vi "TDMS Advanced - Write Synchronously.vi"   [LabVIEW 2020]
panel:
  # "For instructions, select Help>>Show Context Help and move the cursor over the VI icon to display help for this VI."
types:
  T1 = enum16{"open", "open or create", "create or replace", "create", "open (read-only)"}
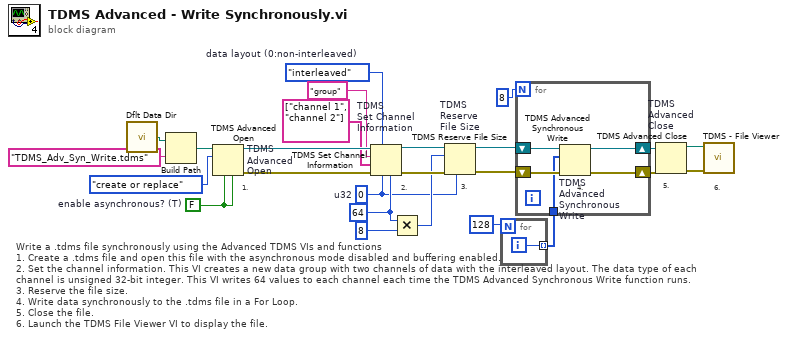
[diagram p0: block diagram]
diagram:
  w3 = FALSE  # enable asynchronous? (T)
  w7 = u32 64 ("samples per channel")
  w4 = u32 0  # u32
  w17 = enum16{"non-interleaved", "interleaved"}."interleaved"  # data layout (0:non-interleaved)
  # "Write a .tdms file synchronously using the Advanced TDMS VIs and functions\n1. Create a .tdms file and open this file with the asynchronous mode disabled and buffering enabled.\n2. Set the channel information. This VI creates a new data group with two channels of data with the interleaved layout. The data type of each channel is unsigned 32-bit integer. This VI writes 64 values to each channel each time the TDMS Advanced Synchronous Write function runs.\n3. Reserve the file size.\n4. Write data synchronously to the .tdms file in a For Loop.\n5. Close the file.\n6. Launch the TDMS File Viewer VI to display the file."
  # "6."
  # "1."
  # "5."
  # "3."
  # "2."
  n1 = call <vilib>:"Dflt Data Dir.vi"() -> ("App:Default Data Directory"=w20:path)
  n2 = Build Path(base path=w20, name or relative path="TDMS_Adv_Syn_Write.tdms") -> (appended path=w24:path)
  n3 = TDMS Advanced Open "TDMS\nAdvanced\nOpen"(4:w3, 6:w3, 10:T1."create or replace" ("operation (0:open)"), 11:w24) -> (0:w22:errorcluster, 3:w21:refnum<k34>)  [unwired: 1 in, 1 out]
  n4 = TDMS Set Channel Information "TDMS\nSet Channel\nInformation"(4:w7, 6:w4, 7:w17, 8:w22, 9:string[] ["channel 1", "channel 2"] ("channel name(s)"), 10:"group" ("group name (Untitled)"), 11:w21) -> (0:w9:errorcluster, 3:w8:refnum<k34>)
  n5 = Multiply(x=w7, y=u32 8) -> (x*y=w5:u32)
  n6 = TDMS Reserve File Size "TDMS\nReserve\nFile Size"(6:w4, 8:w9, 10:w5, 11:w8) -> (0:w11:errorcluster, 3:w10:refnum<k34>)  [unwired: 1 in]
  n7 = for {
    N: 128 -> [_]
    tunnel: [w26] -> w14 mode=indexing
    i -> [w26]
  }
  n8 = for {
    N: 8 -> [_]
    shift-right: [w28] -> w12
    shift-left: w10 -> [w30]
    shift-right: [w29] -> w13
    shift-left: w11 -> [w31]
    tunnel: w14 -> [w27]
    # "4."
    n9 = TDMS Advanced Synchronous Write "TDMS\nAdvanced\nSynchronous\nWrite"(8:w31, 10:w27, 11:w30) -> (0:w29:errorcluster, 3:w28:refnum<k34>)
  }
  n10 = TDMS Advanced Close "TDMS\nAdvanced\nClose"(8:w13, 11:w12) -> (0:w2:errorcluster, 3:w1:path)  [unwired: 2 in]
  n11 = call <vilib>:"TDMS - File Viewer.vi"("error in (no error)"=w2, "file path"=w1) -> ()  [unwired: 4 in, 2 out]
